vi "Temperature Multiplot.vi"() -> ()   [LabVIEW 2014]
doc: "This VI is the solution to an exercise in the LabVIEW Core I course.\n\nIt is used to demonstrate While loops and waveform charts. This VI simulates a temperature reading once every 500 ms and plots the data in a strip chart."
panel:
  out "Average Temperature History":cluster{dbl, "Temperature":dbl}(graph)
  in  "Power":bool=TRUE
  # "The Temperature Monitor VI acquires and displays temperature. Modify the VI to average the last five\ntemperature measurements and display the running average on the waveform chart."
  # "ON\n\nOFF"
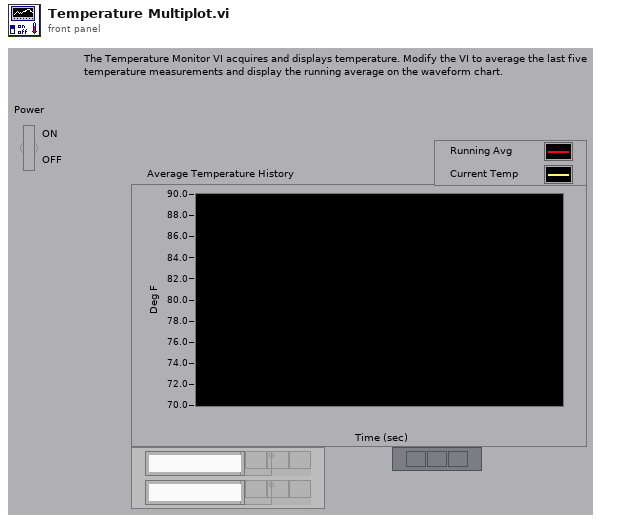
[diagram p1: front panel]
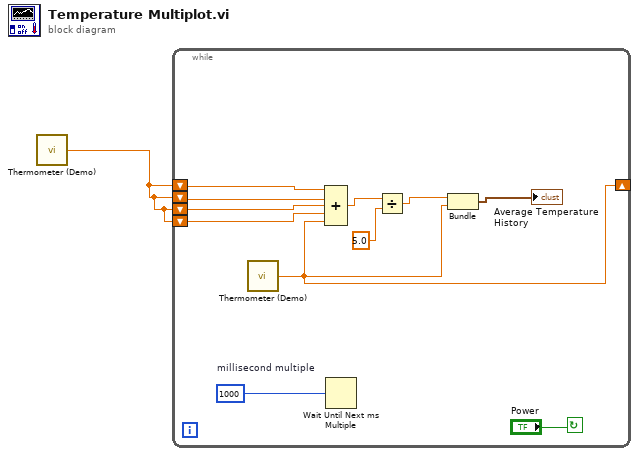
[diagram p0: block diagram]
diagram:
  n1 = call "Thermometer (Demo).vi"() -> ("Temperature"=w1:dbl)  [unwired: 1 in]
  n2 = while {
    shift-right: [w3] -> _
    shift-left: w1 -> [w10]
    shift-left: w1 -> [w7]
    shift-left: w1 -> [w8]
    shift-left: w1 -> [w9]
    stop <- "Power" continue-if-true
    w11 = u32 1000  # millisecond multiple
    n3 = call "Thermometer (Demo).vi"() -> ("Temperature"=w3:dbl)  [unwired: 1 in]
    n4 = Compound Arithmetic op=ADD(w10, w9, w8, w7, w3) -> (w6:dbl)
    n5 = Wait Until Next ms Multiple(millisecond multiple=w11) -> ()  [unwired: 1 out]
    n6 = Divide(x=w6, y=5.0) -> (x/y=w4:dbl)
    n7 = Bundle(w4, "Temperature"=w3) -> (→"Average Temperature History":cluster{dbl, "Temperature":dbl})  [unwired: 1 in]
  }
